vi "grayscale-convert.vi"(9 "B":u8, 10 "G":u8, 11 "R":u8) -> (3 "Output pixel":dbl)   [LabVIEW 2021]
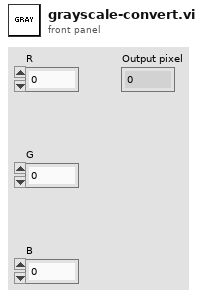
[diagram p1: front panel]
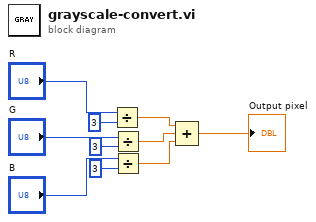
[diagram p0: block diagram]
diagram:
  n1 = Divide(x="R", y=u8 3) -> (x/y=w7:dbl)
  n2 = Divide(x="G", y=u8 3) -> (x/y=w8:dbl)
  n3 = Divide(x="B", y=u8 3) -> (x/y=w9:dbl)
  n4 = Compound Arithmetic op=ADD(w7, w8, w9) -> (→"Output pixel":dbl)
